vi "log.vi"(8 "error in (no error)":errorcluster, 10 "log_entry":T1 {"datetime" format="%<%x %.3X>T"}, 11 "json.provider in":refnum<class "json.provider.lvclass">) -> (0 "error out":errorcluster, 3 "json.provider out":refnum<class "json.provider.lvclass">)   [LabVIEW 2021, in "json.provider.lvclass"]
uses:
  json.provider.lvclass
  Z:/Projects/DIT/lv-default-repo/source/system.logging.provider/system.logging.provider.lvclass
  system.logging/log_entry.ctl
  system.logging/severity.ctl
  system.logging.provider.lvclass/system.logging.provider.ctl
  json.provider.lvclass/json.provider.ctl
  system.logging.provider.lvclass
  system.logging/system.logging.lvclass
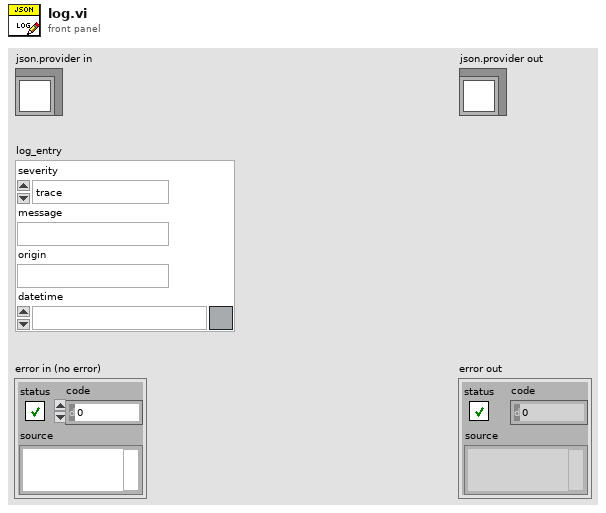
[diagram p1: front panel]
types:
  T1 = typedef "system.logging.lvclass/log_entry.ctl" = cluster{"severity":T2, "message":string, "origin":string, "datetime":timestamp}
  T2 = typedef "system.logging.lvclass/severity.ctl" = enum8{"trace", "debug", "info", "warning", "error"}
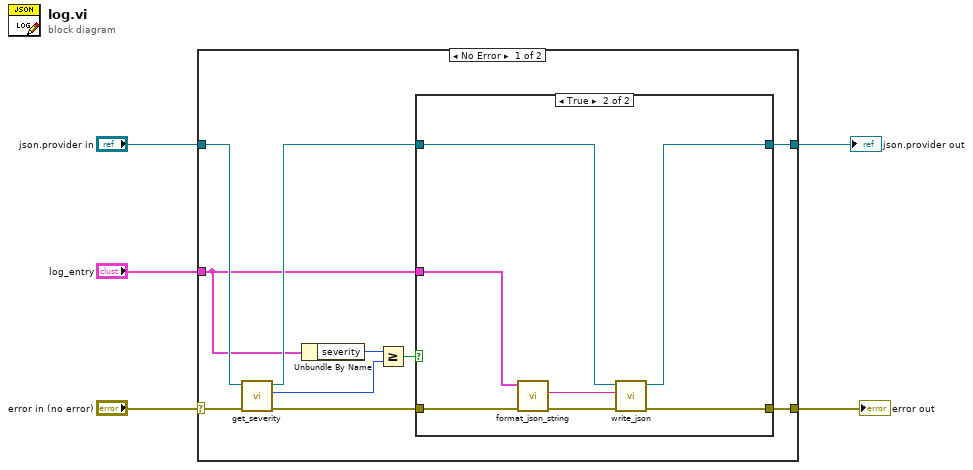
[diagram p0: block diagram]
diagram:
  n1 = case shown="No Error" "error in (no error)" {
    selector: "error in (no error)" -> [w15 w26]
    tunnel: [w8 w26] -> w2
    tunnel: [w7 w25] -> w1
    tunnel: "json.provider in" -> [w14 w25]
    tunnel: "log_entry" -> [w6 _]
    frame No Error {
      n2 = call "get_severity.vi"("error in (no error)"=w15, "system.logging.provider in"=w14) -> ("error out"=w10:errorcluster, "severity"=w12:T2, "system.logging.provider out"=w9:refnum<class "json.provider.lvclass">)  [unwired: 7 in]
      n3 = Unbundle By Name(w6) -> ("severity"=w13:T2)
      n4 = Greater Or Equal?(x=w13, y=w12) -> (x >= y?=w11:bool)
      n5 = case shown="True" w11 {
        tunnel: w10 -> [w17 w24]
        tunnel: w9 -> [w16 w20]
        tunnel: [w17 w21] -> w8
        tunnel: [w16 w19] -> w7
        tunnel: w6 -> [_ w23]
        frame False {
          # "Discard, entry"
        }
        frame True {
          n6 = call "format_json_string.vi"("error in (no error)"=w24, "log_entry"=w23) -> ("error out"=w22:errorcluster, "json"=w18:string)  [unwired: 8 in]
          n7 = call "write_json.vi"("error in (no error)"=w22, "json"=w18, "json.provider in"=w20) -> ("error out"=w21:errorcluster, "json.provider out"=w19:refnum<class "json.provider.lvclass">)  [unwired: 7 in]
        }
      }
    }
    frame Error {
    }
  }
  "error out" <- w2
  "json.provider out" <- w1
